vi "relativeMove.vi"(7 "模式":enum16{"快速移动", "规划速度"}(ring), 8 "错误输入":errorcluster, 9 "Param_StepDis":dbl, 10 "TargetY":dbl, 11 "TargetX":dbl) -> (0 "错误输出":errorcluster)   [LabVIEW 2011]
uses:
  API/API DYM.lvlib
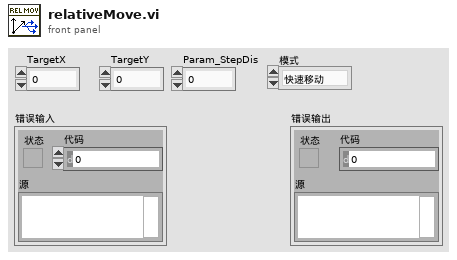
[diagram p1: front panel]
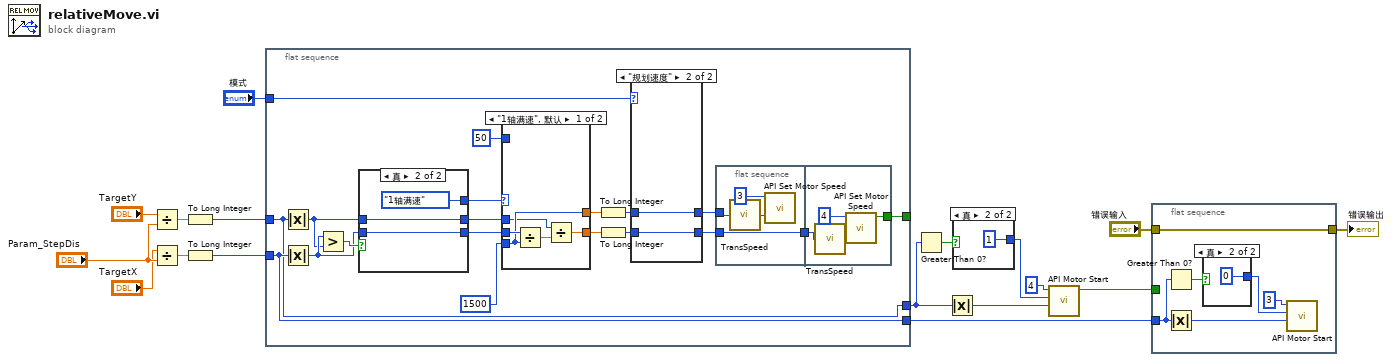
[diagram p0: block diagram]
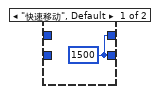
[diagram p2: hidden frame]
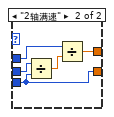
[diagram p3: hidden frame]
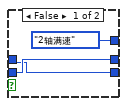
[diagram p4: hidden frame]
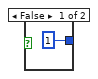
[diagram p5: hidden frame]
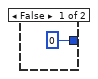
[diagram p6: hidden frame]
diagram:
  n1 = Divide(x="TargetY", y="Param_StepDis") -> (x/y=w16:dbl)
  n2 = Divide(x="TargetX", y="Param_StepDis") -> (x/y=w11:dbl)
  n3 = To Long Integer(number=w16) -> (32bit integer=w8:i32)
  n4 = To Long Integer(number=w11) -> (32bit integer=w10:i32)
  n5 = flat-sequence {
    tunnel: w10 -> [w36]
    tunnel: [w36] -> w9
    tunnel: w8 -> [w35]
    tunnel: [w35] -> w7
    tunnel: "模式" -> [w24]
    tunnel: [w18] -> _
    frame #0 {
      n6 = Absolute Value(x=w35) -> (abs(x)=w29:i32)
      n7 = Absolute Value(x=w36) -> (abs(x)=w30:i32)
      n8 = Greater?(x=w30, y=w29) -> (0:w34:bool)
      n9 = case shown="真" w34 {
        tunnel: [enum16{"1轴满速", "2轴满速"}."2轴满速" enum16{"1轴满速", "2轴满速"}."1轴满速"] -> w33
        tunnel: w30 -> [w59 w62]
        tunnel: w29 -> [w58 w61]
        tunnel: [w58 w62] -> w28
        tunnel: [w59 w61] -> w27
        frame False {
        }
        frame True {
        }
      }
      n10 = case shown="\"1轴满速\", 默认" w33 {
        tunnel: 1500 -> [w50 w56]
        tunnel: 50 -> [_ _]
        tunnel: w28 -> [w52 w57]
        tunnel: w27 -> [w49 w54]
        tunnel: [w50 w53] -> w25
        tunnel: [w48 w56] -> w26
        frame "1轴满速", Default {
          n11 = Divide(x=w52, y=w50) -> (x/y=w51:dbl)
          n12 = Divide(x=w49, y=w51) -> (x/y=w48:dbl)
        }
        frame "2轴满速" {
          n13 = Divide(x=w57, y=w56) -> (x/y=w55:dbl)
          n14 = Divide(x=w54, y=w55) -> (x/y=w53:dbl)
        }
      }
      n15 = To Long Integer(number=w25) -> (32bit integer=w23:i32)
      n16 = To Long Integer(number=w26) -> (32bit integer=w22:i32)
      n17 = case shown="\"规划速度\"" w24 {
        tunnel: w23 -> [_ w38]
        tunnel: w22 -> [_ w39]
        tunnel: [w37 w39] -> w20
        tunnel: [w37 w38] -> w21
        frame "快速移动", Default {
          w37 = 1500
        }
        frame "规划速度" {
        }
      }
      n18 = flat-sequence {
        tunnel: w21 -> [w41]
        tunnel: w20 -> [w42]
        tunnel: [w42] -> w19
        tunnel: w19 -> [w45]
        tunnel: [w46] -> w18
        frame #0 {
          n19 = call "TransSpeed.vi"("Speed_In"=w41) -> ("Speed_Out"=w40:i32)
          n20 = call "API Set Motor Speed.vi"("motorSpeed"=w40, "motorNum"=3) -> ()  [unwired: 9 in, 1 out]
        }
        frame #1 {
          n21 = call "TransSpeed.vi"("Speed_In"=w45) -> ("Speed_Out"=w44:i32)
          n22 = call "API Set Motor Speed.vi"("motorSpeed"=w44, "motorNum"=4) -> ("setmotorspeed return value"=w46:bool)  [unwired: 9 in]
        }
      }
    }
  }
  n23 = Greater Than 0?(x=w7) -> (x > 0?=w15:bool)
  n24 = Absolute Value(x=w7) -> (abs(x)=w6:i32)
  n25 = case shown="真" w15 {
    tunnel: [0 1] -> w14
    frame False {
    }
    frame True {
    }
  }
  n26 = call "API Motor Start.vi"("stepNum"=w6, "direction"=w14, "motorNum"=4) -> ("motorStart return value"=w13:bool)  [unwired: 8 in]
  n27 = flat-sequence {
    tunnel: w13 -> [_]
    tunnel: "错误输入" -> [w66]
    tunnel: w9 -> [w68]
    tunnel: [w66] -> w5
    frame #0 {
      n28 = Greater Than 0?(x=w68) -> (x > 0?=w71:bool)
      n29 = Absolute Value(x=w68) -> (abs(x)=w67:i32)
      n30 = case shown="真" w71 {
        tunnel: [1 0] -> w70
        frame False {
        }
        frame True {
        }
      }
      n31 = call "API Motor Start.vi"("stepNum"=w67, "direction"=w70, "motorNum"=3) -> ()  [unwired: 8 in, 1 out]
    }
  }
  "错误输出" <- w5
